vi "InitializeOpStates.vi"(7 "op state defs":T1[](array[typedef]), 9 "metric ids":string[](array[string]), 10 "data group name":string, 11 "operating states in":T6[](array[typedef])) -> (1 "valid config":bool, 3 "sorted operating states":T2[](array[typedef]))   [LabVIEW 2017, in "OpState.lvlib"]
uses:
  <vilib>/addons/InsightCM/Devices/Shared/Common/OpState/OpState.lvlib
  <vilib>/addons/InsightCM/MessageBus/Base/controls/OperatingState.ctl
  <vilib>/addons/InsightCM/MessageBus/Base/controls/KeyValuePair.ctl
  <vilib>/addons/InsightCM/MessageBus/Base/controls/Trigger.ctl
  <vilib>/addons/InsightCM/MessageBus/Base/controls/Condition.ctl
  <vilib>/addons/InsightCM/Devices/Shared/Common/OpState/controls/TriggerOperatingState.ctl
  <vilib>/addons/InsightCM/Devices/Shared/Common/Trigger/controls/TriggerCondition.ctl
  <vilib>/addons/InsightCM/MessageBus/Base/controls/ConfigListItem.ctl
  <vilib>/addons/InsightCM/Utilities/DeviceModelHelpers/DeviceModelHelpers.lvlib
  <vilib>/addons/InsightCM/Devices/Shared/Common/Trigger/Trigger.lvlib
  <vilib>/addons/InsightCM/Utilities/PropertyHelpers/PropertyHelpers.lvlib
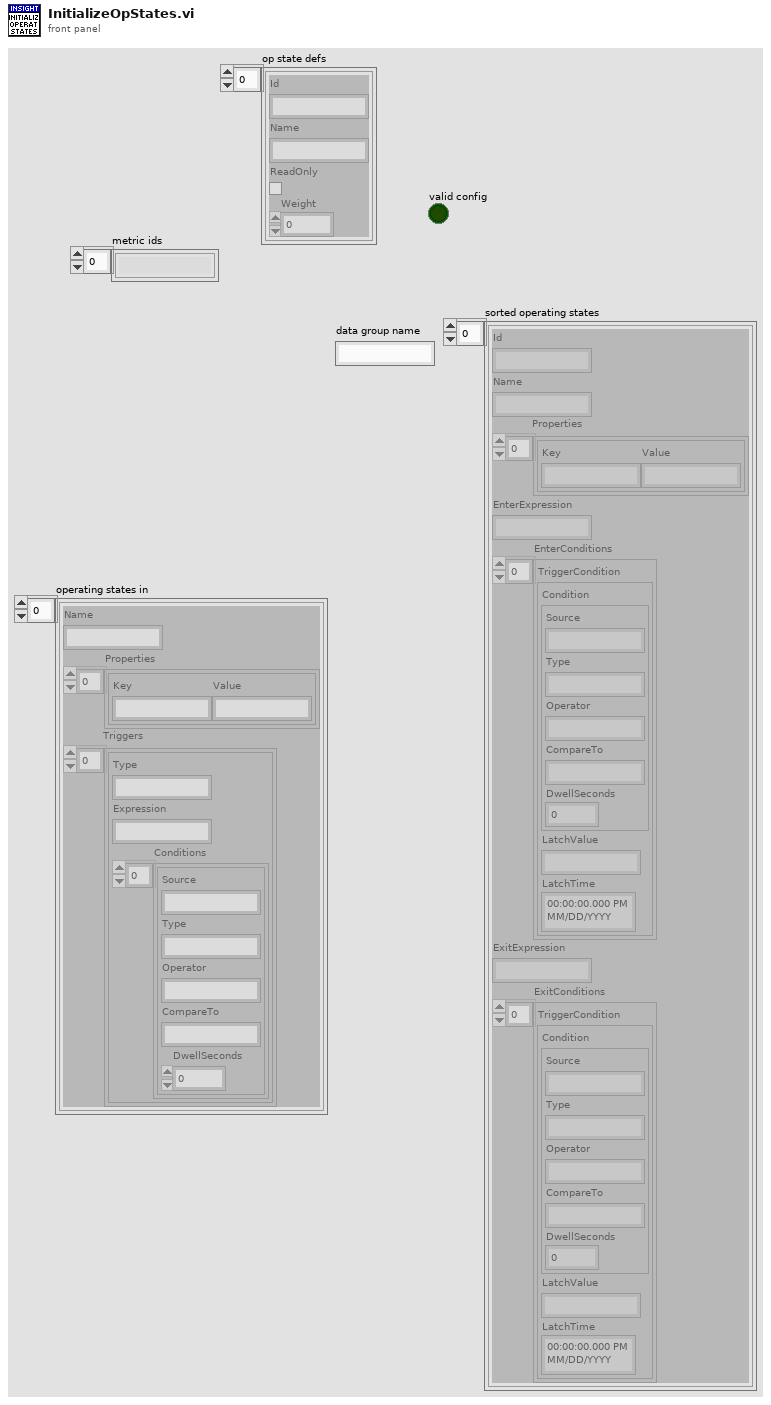
[diagram p1: front panel]
types:
  T1 = typedef "ConfigListItem.ctl" = cluster{"Id":string, "Name":string, "ReadOnly":bool, "Weight":i32}
  T2 = typedef "OpState.lvlib/TriggerOperatingState.ctl" = cluster{"Id":string, "Name":string, "Properties":T3[], "EnterExpression":string, "EnterConditions":T4[], "ExitExpression":string, "ExitConditions":T4[]}
  T3 = typedef "KeyValuePair.ctl" = cluster{"Key":string, "Value":string}
  T4 = typedef "Trigger.lvlib/TriggerCondition.ctl" = cluster{"Condition":T5, "LatchValue":string, "LatchTime":timestamp}
  T5 = typedef "Condition.ctl" = cluster{"Source":string, "Type":string, "Operator":string, "CompareTo":string, "DwellSeconds":dbl}
  T6 = typedef "OperatingState.ctl" = cluster{"Name":string, "Properties":T3[], "Triggers":T7[]}
  T7 = typedef "Trigger.ctl" = cluster{"Type":string, "Expression":string, "Conditions":T5[]}
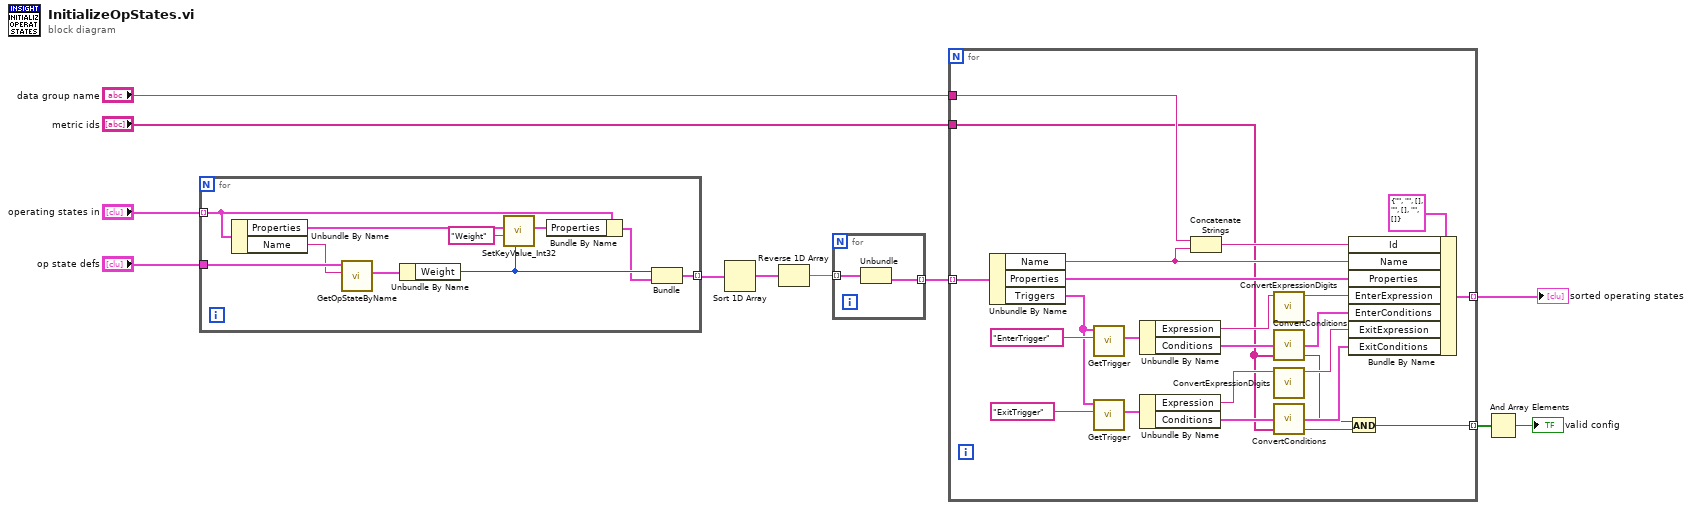
[diagram p0: block diagram]
diagram:
  n1 = for {
    tunnel: "operating states in" -> [w17] mode=indexing
    tunnel: "op state defs" -> [w21]
    tunnel: [w18] -> w3 mode=indexing
    n2 = Unbundle By Name(w17) -> ("Properties"=w15:T3[], "Name"=w20:string)
    n3 = call <vilib>:"GetOpStateByName.vi"("name"=w20, "op state defs in"=w21) -> ("op state"=w19:T1)  [unwired: 7 in, 2 out]
    n4 = Unbundle By Name(w19) -> ("Weight"=w13:i32)
    n5 = call <vilib>:"SetKeyValue_Int32.vi"("value"=w13, "key"="Weight", "key value pairs"=w15) -> ("key value pairs out"=w16:T3[])  [unwired: 8 in]
    n6 = Bundle By Name(cluster=w17, "Properties"=w16) -> (w12:T6)
    n7 = Bundle("Weight"=w13, "OperatingState 2"=w12) -> (w18:cluster{"Weight":i32, "OperatingState 2":T6})  [unwired: 1 in]
  }
  n8 = Sort 1D Array(array=w3) -> (sorted array=w2:cluster{"Weight":i32, "OperatingState 2":T6}[])
  n9 = Reverse 1D Array(array=w2) -> (reversed array=w1:cluster{"Weight":i32, "OperatingState 2":T6}[])
  n10 = for {
    tunnel: w1 -> [w23] mode=indexing
    tunnel: [w22] -> w10 mode=indexing
    n11 = Unbundle(w23) -> ("OperatingState 2"=w22:T6)  [unwired: 1 out]
  }
  n12 = for {
    tunnel: w10 -> [w47] mode=indexing
    tunnel: [w45] -> w9 mode=indexing
    tunnel: "data group name" -> [w42]
    tunnel: "metric ids" -> [w27]
    tunnel: [w24] -> w6 mode=indexing
    n13 = Unbundle By Name(w47) -> ("Name"=w44:string, "Properties"=w41:T3[], "Triggers"=w33:T7[])
    n14 = call <vilib>:"GetTrigger.vi"("type"="EnterTrigger", "triggers"=w33) -> ("trigger"=w39:T7)  [unwired: 8 in, 1 out]
    n15 = call <vilib>:"GetTrigger.vi"("type"="ExitTrigger", "triggers"=w33) -> ("trigger"=w34:T7)  [unwired: 8 in, 1 out]
    n16 = Unbundle By Name(w39) -> ("Expression"=w31:string, "Conditions"=w38:T5[])
    n17 = Unbundle By Name(w34) -> ("Expression"=w29:string, "Conditions"=w35:T5[])
    n18 = Concatenate Strings(w42, w44) -> (w43:string)
    n19 = call <vilib>:"ConvertExpressionDigits.vi"("input"=w31) -> ("output"=w30:string)  [unwired: 10 in]
    n20 = call <vilib>:"ConvertConditions.vi"("metric ids"=w27, "conditions"=w38) -> ("valid config"=w26:bool, "trigger conditions"=w37:T4[])  [unwired: 2 in]
    n21 = call <vilib>:"ConvertExpressionDigits.vi"("input"=w29) -> ("output"=w28:string)  [unwired: 10 in]
    n22 = call <vilib>:"ConvertConditions.vi"("metric ids"=w27, "conditions"=w35) -> ("valid config"=w25:bool, "trigger conditions"=w36:T4[])  [unwired: 2 in]
    n23 = Bundle By Name(cluster=T2 {"Id"="", "Name"="", "Properties"=[], "EnterExpression"="", "EnterConditions"=[], "ExitExpression"="", "ExitConditions"=[]} ("OperatingState"), "Id"=w43, "Name"=w44, "Properties"=w41, "EnterExpression"=w30, "EnterConditions"=w37, "ExitExpression"=w28, "ExitConditions"=w36) -> (w45:T2)
    n24 = And(x=w26, y=w25) -> (x .and. y?=w24:bool)
  }
  "sorted operating states" <- w9
  n25 = And Array Elements(Boolean array=w6) -> (logical AND=→"valid config":bool)
